vi "Block Float (I32).vi"(8 "Input Valid":bool=TRUE, 10 "Binary Number 2":i32 format="%032b", 11 "Binary Number 1":i32 format="%032b") -> (0 "Output Valid":bool=TRUE, 2 "Block Float Mantissa 2":i32 format="%032b", 3 "Block Float Mantissa 1":i32 format="%032b", 5 "Common Exponent":i8)   [LabVIEW 2010]
doc: "This VI computes the block floating point representation of two numbers"
panel:
  out "shifted number2":fxp<+/-,32,1> format="%.32g"
  out "shifted number1":fxp<+/-,32,1> format="%.32g"
  out "number 2":fxp<+/-,32,1> format="%.32g"
  out "number1":fxp<+/-,32,1> format="%.32g"
  # "n1=0.5, n2=.25\nn1=-0.375, n2=-0.75"
  # "Check:\na) If Input1=0\nb)If Input2=0\nc)If Input1 and2=0\nd)If Input1 and 2!=0\ne)If Input2 =-1"
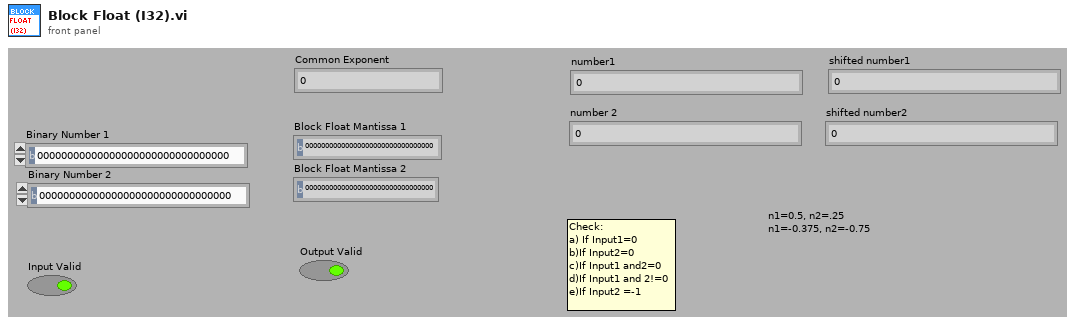
[diagram p1: front panel]
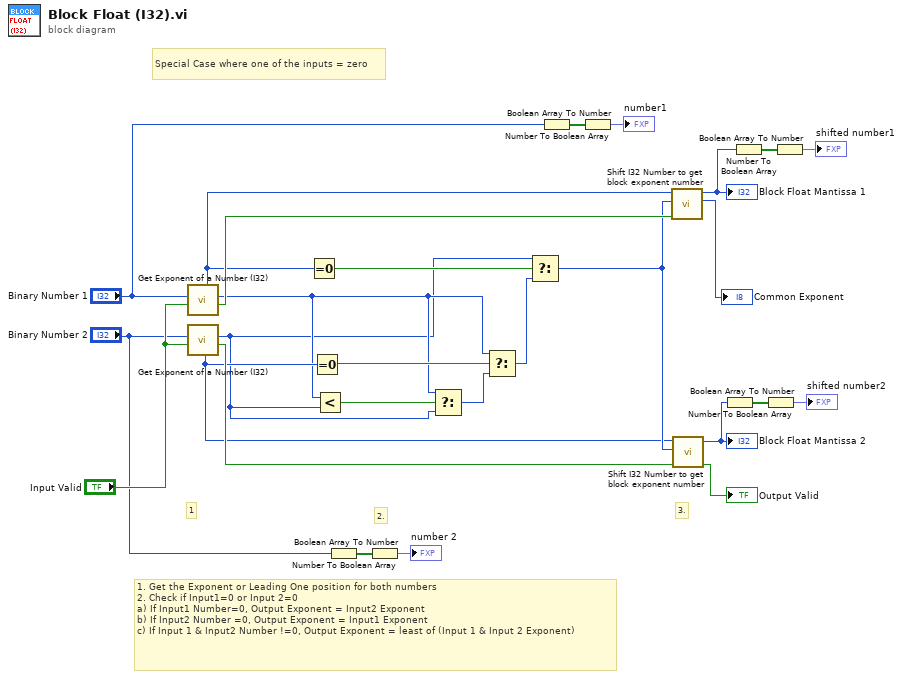
[diagram p0: block diagram]
diagram:
  # "1. Get the Exponent or Leading One position for both numbers\n2. Check if Input1=0 or Input 2=0\na) If Input1 Number=0, Output Exponent = Input2 Exponent\nb) If Input2 Number =0, Output Exponent = Input1 Exponent\nc) If Input 1 & Input2 Number !=0, Output Exponent = least of (Input 1 & Input 2 Exponent)"
  # "3."
  # "2."
  # "1"
  # "Special Case where one of the inputs = zero"
  n1 = call "Get Exponent of a Number (I32).vi"("Input Valid"="Input Valid", "Binary Number"="Binary Number 1") -> ("Output Valid"=w26:bool, "Exponent"=w15:u8, "Binary Number"=w17:i32)  [unwired: 7 in]
  n2 = call "Get Exponent of a Number (I32).vi"("Input Valid"="Input Valid", "Binary Number"="Binary Number 2") -> ("Output Valid"=w27:bool, "Exponent"=w1:u8, "Binary Number"=w16:i32)  [unwired: 7 in]
  n3 = Equal To 0?(x=w17) -> (x = 0?=w22:bool)
  n4 = Equal To 0?(x=w16) -> (x = 0?=w21:bool)
  n5 = Less?(x=w15, y=w1) -> (x < y?=w23:bool)
  n6 = Number To Boolean Array(number="Binary Number 2") -> (Boolean array=w10:bool[])
  n7 = Boolean Array To Number(Boolean array=w10) -> (number=→"number 2":fxp<+/-,32,1>)
  n8 = Select(t=w15, s=w23, f=w1) -> (s? t:f=w2:u8)
  n9 = Select(t=w15, s=w21, f=w2) -> (s? t:f=w20:u8)
  n10 = Select(t=w1, s=w22, f=w20) -> (s? t:f=w19:u8)
  n11 = Number To Boolean Array(number="Binary Number 1") -> (Boolean array=w14:bool[])
  n12 = Boolean Array To Number(Boolean array=w14) -> (number=→"number1":fxp<+/-,32,1>)
  n13 = call "Shift I32 Number to get block exponent number.vi"("Input Valid"=w26, "Leading Zero Position"=w19, "Binary Number"=w17) -> ("Block Float Exponent"=→"Common Exponent":i8, "Block Float Mantissa"=w6:i32)  [unwired: 6 in, 1 out]
  "Block Float Mantissa 1" <- w6
  n14 = call "Shift I32 Number to get block exponent number.vi"("Input Valid"=w27, "Leading Zero Position"=w19, "Binary Number"=w16) -> ("Output Valid"=→"Output Valid":bool, "Block Float Mantissa"=w3:i32)  [unwired: 6 in, 1 out]
  "Block Float Mantissa 2" <- w3
  n15 = Number To Boolean Array(number=w3) -> (Boolean array=w5:bool[])
  n16 = Number To Boolean Array(number=w6) -> (Boolean array=w7:bool[])
  n17 = Boolean Array To Number(Boolean array=w5) -> (number=→"shifted number2":fxp<+/-,32,1>)
  n18 = Boolean Array To Number(Boolean array=w7) -> (number=→"shifted number1":fxp<+/-,32,1>)
